vi "Do.vi"(8 "error in (no error)":errorcluster, 9 "Events":refnum<class "Events.lvclass">, 10 "Message Loop Data in":T1, 11 "IInternalRequest in":refnum<class "IHandlePublished.lvclass">) -> (0 "error out":errorcluster, 2 "Message Loop Data out":T1, 3 "IInternalRequest out":refnum<class "IHandlePublished.lvclass">)   [LabVIEW 2020, in "wamplv.lvlib" / "IHandlePublished.lvclass"]
uses:
  IHandlePublished.lvclass
  Publish/IPublish/IPublish.lvclass
  WAMP Client/Private/TypeDef/Publish Requests Map.ctl
  wamplv.lvlib
  WAMP Client/Private/TypeDef/Endpoint Data.ctl
  Call/ICallRequest/ICallRequest.lvclass
  WAMP Client/Private/TypeDef/CALL Request Map.ctl
  WAMP Client/Private/TypeDef/SUBSCRIBE Requests Map.ctl
  WAMP Client/Private/TypeDef/Subscriptions Map.ctl
  WAMP Client/Private/TypeDef/Unsubscribe Requests Map.ctl
  WAMP Client/Private/TypeDef/Unregister requests map.ctl
  WAMP Client/Private/TypeDef/Message Loop Data.ctl
  Events/EventsParent/Events.lvclass
  Subscribe/ISubscribe/ISubscribe.lvclass
  Message loop classes/Subscription details/SubscriptionDetailsParent/SubscriptionDetailsParent.lvclass
  Unsubscribe/IUnsubscribe/IUnsubscribe.lvclass
  Register/IRegister/IRegister.lvclass
  Unregister/IUnregister/IUnregister.lvclass
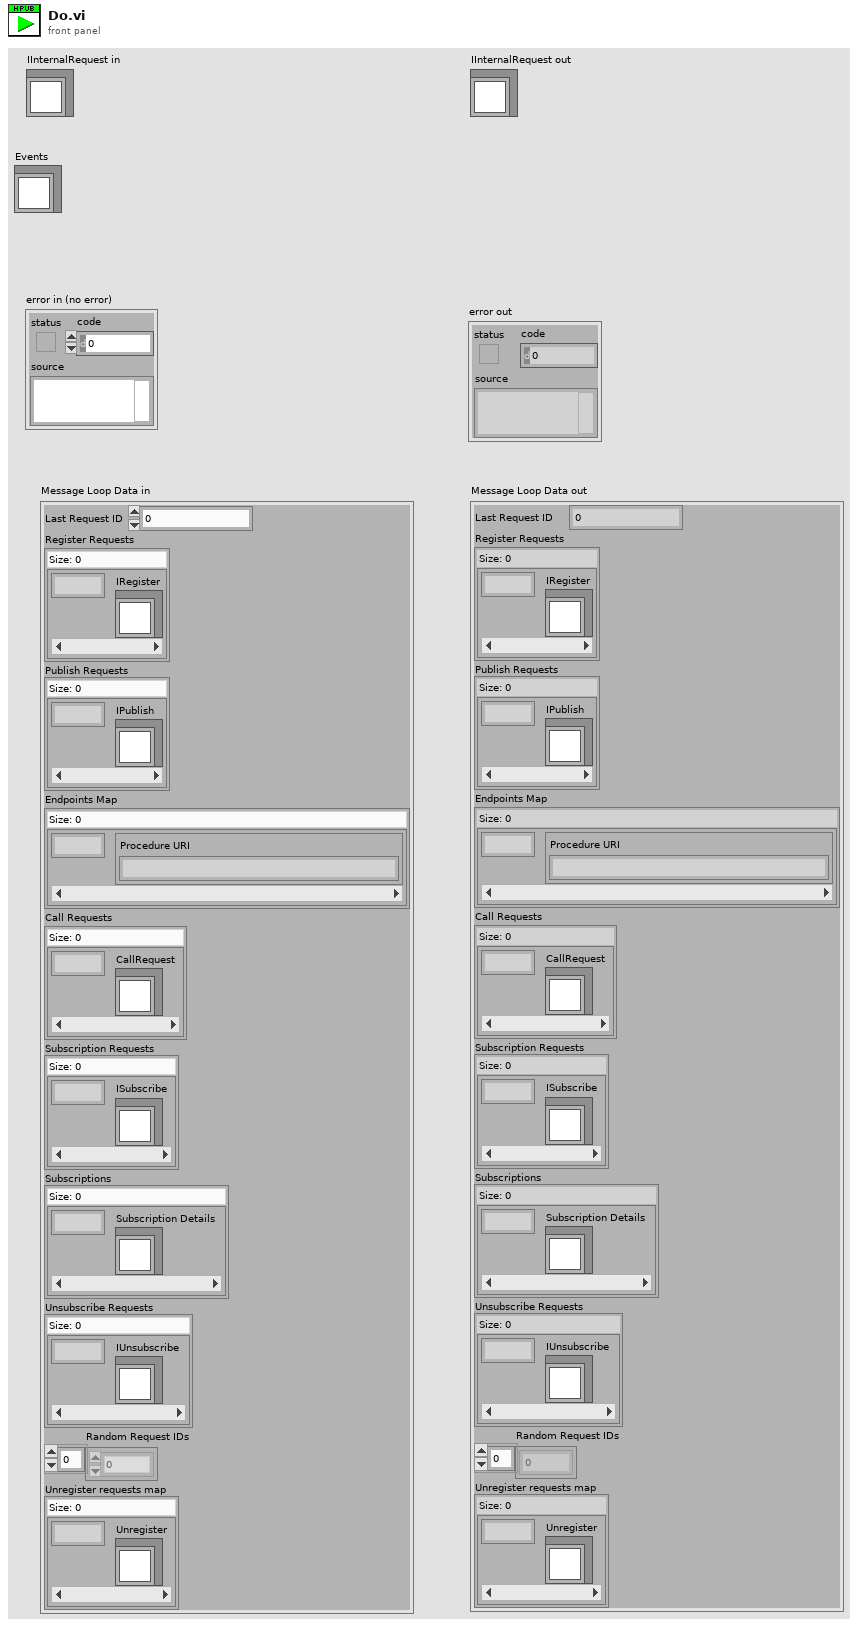
[diagram p1: front panel]
types:
  T1 = typedef "wamplv.lvlib/Message Loop Data.ctl" = cluster{"Last Request ID":u64, "Register Requests":map{u64, refnum<class "IRegister.lvclass">}, "Publish Requests":T2, "Endpoints Map":map{u64, T3}, "Call Requests":T4, "Subscription Requests":T5, "Subscriptions":T6, "Unsubscribe Requests":T7, "Random Request IDs":u64[], "Unregister requests map":T8}
  T2 = typedef "wamplv.lvlib/Publish Requests Map.ctl" = map{u64, refnum<class "IPublish.lvclass">}
  T3 = typedef "wamplv.lvlib/Endpoint Data.ctl" = cluster{"Procedure URI":string}
  T4 = typedef "wamplv.lvlib/CALL Request Map.ctl" = map{u64, refnum<class "ICallRequest.lvclass">}
  T5 = typedef "wamplv.lvlib/SUBSCRIBE Requests Map.ctl" = map{u64, refnum<class "ISubscribe.lvclass">}
  T6 = typedef "wamplv.lvlib/Subscriptions Map.ctl" = map{u64, refnum<class "SubscriptionDetailsParent.lvclass">}
  T7 = typedef "wamplv.lvlib/Unsubscribe Requests Map.ctl" = map{u64, refnum<class "IUnsubscribe.lvclass">}
  T8 = typedef "wamplv.lvlib/Unregister requests map.ctl" = map{u64, refnum<class "IUnregister.lvclass">}
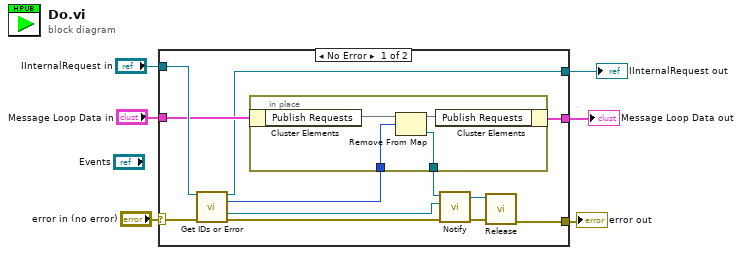
[diagram p0: block diagram]
diagram:
  n1 = case shown="No Error" "error in (no error)" {
    selector: "error in (no error)" -> [w17 w25]
    tunnel: "IInternalRequest in" -> [w18 w23]
    tunnel: "Message Loop Data in" -> [w15 w24]
    tunnel: [w14 w24] -> w3
    tunnel: [w13 w23] -> w2
    tunnel: [w7 w25] -> w1
    frame No Error {
      n2 = call-dynamic "Get IDs or Error.vi"("IHandlePublished in"=w18, "error in (no error)"=w17) -> ("IHandlePublished out"=w13:refnum<class "IHandlePublished.lvclass">, "Publish request ID"=w16:u64, "ErrorOrSuccess"=w10:refnum<class "ErrorOrSuccess.lvclass">, "error out"=w11:errorcluster)  [unwired: 9 in, 1 out]
      n3 = in-place "In Place Element Structure" {
        in-place-border: w16 -> [w22]
        in-place-border: [w19] -> w12
        n4 = in-place-cluster #1(w15) -> ("Publish Requests"=w21:T2)
        n5 = Remove From Map(10:w22, 11:w21) -> (1:w19:refnum<class "IPublish.lvclass">, 3:w20:T2)  [unwired: 1 out]
        n6 = in-place-cluster #1("Publish Requests"=w20) -> (w14:T1)
      }
      n7 = call-dynamic "Notify.vi"("error in (no error)"=w11, "ErrorOrSuccess"=w10, "IPublish in"=w12) -> ("error out"=w9:errorcluster, "IPublish out"=w8:refnum<class "IPublish.lvclass">)  [unwired: 7 in]
      n8 = call-dynamic "Release.vi"("error in (no error)"=w9, "IContainersNotiferOrEvents in"=w8) -> ("error out"=w7:errorcluster)  [unwired: 9 in]
    }
    frame Error {
    }
  }
  "error out" <- w1
  "IInternalRequest out" <- w2
  "Message Loop Data out" <- w3
